vi "LEDExecute.vi"   [LabVIEW 2023]
uses:
  <vilib>/Rock Robotics/WPI/DriverStation/WPI_DriverStationAllianceInfo.ctl
  Intake/IntakeGlobal.vi
types:
  T1 = typedef "WPI_DriverStationAllianceInfo.ctl" = enum16{"Red", "Blue", "Invalid"}
  T2 = typedef "WPI_DigitalOutputDevRef.ctl" = cluster{"DIO Channel":T3, "DevStatus":errorcluster}
  T3 = typedef "FPGA_DIOChannel.ctl" = enum8{"DIO 0", "DIO 1", "DIO 2", "DIO 3", "DIO 4", "DIO 5", "DIO 6", "DIO 7", "DIO 8", "DIO 9", "DIO MXP 0", "DIO MXP 1", "DIO MXP 2", "DIO MXP 3", "DIO MXP 4", "DIO MXP 5", "DIO MXP 6", "DIO MXP 7", "DIO MXP 8", "DIO MXP 9", "DIO MXP 10", "DIO MXP 11", "DIO MXP 12", "DIO MXP 13", "DIO MXP 14", "DIO MXP 15", "SPI Port CS1", "SPI Port CS2", "SPI Port CS3", "SPI Port MISO", "SPI Port MOSI", "Invalid"}
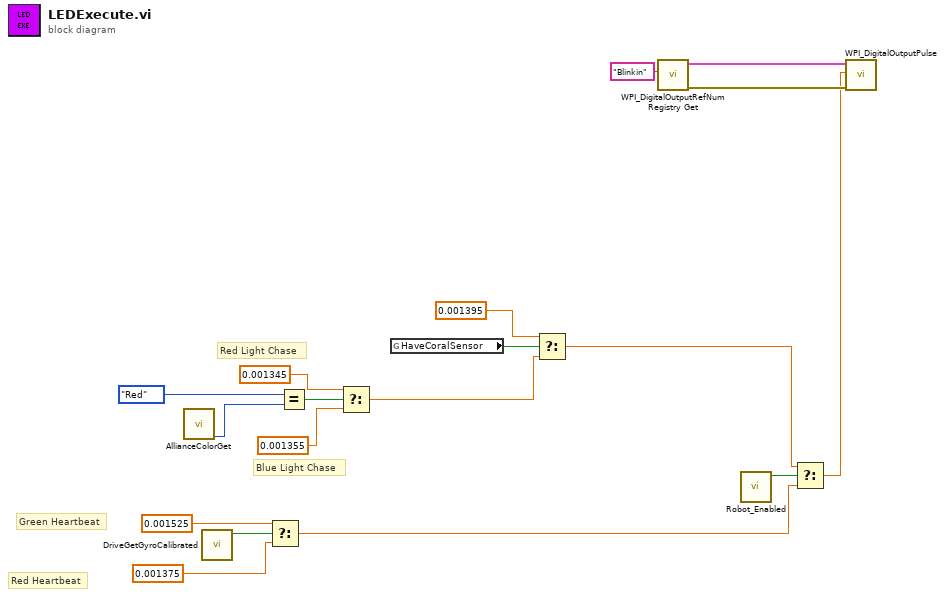
[diagram p0: block diagram]
diagram:
  # "Red Light Chase"
  # "Blue Light Chase"
  # "Green Heartbeat"
  # "Red Heartbeat"
  n1 = call "AllianceColorGet.vi"() -> ("AllianceColor"=w11:T1)  [unwired: 11 in]
  n2 = call "DriveGetGyroCalibrated.vi"() -> ("GryoCalibrated"=w10:bool)  [unwired: 11 in]
  n3 = Select(t=0.001525, s=w10, f=0.001375 ("t")) -> (s? t:f=w7:dbl)
  n4 = Equal?(x=WPI_DriverStationAllianceInfo."Red", y=w11) -> (x = y?=w14:bool)
  n5 = Select(t=0.001345, s=w14, f=0.001355) -> (s? t:f=w3:dbl)
  n6 = global read "IntakeGlobal.vi" "HaveCoralSensor"() -> (w4:bool)
  n7 = Select(t=0.001395, s=w4, f=w3) -> (s? t:f=w1:dbl)
  n8 = call <vilib>:"WPI_DigitalOutputRefNum Registry Get.vi"("refnum name"="Blinkin") -> ("error out"=w17:errorcluster, "DigitalOutputDevRef"=w18:T2)  [unwired: 9 in]
  n9 = call "Robot_Enabled.vi"() -> ("Robot Enabled"=w16:bool)  [unwired: 11 in]
  n10 = Select(t=w1, s=w16, f=w7) -> (s? t:f=w6:dbl)
  n11 = call <vilib>:"WPI_DigitalOutputPulse.vi"("error in (no error)"=w17, "length (Sec)"=w6, "DigitalOutputDevRef"=w18) -> ()  [unwired: 7 in, 2 out]
